vi "S2DS_IncorporateUnitsinChannelNames.vi"(5 "User info":string[](array[string]), 9 "All channel parameters (in)":T1 {"Scan parameters"."Y data taking" items=["in both direction", "in up direction only", "in down direction only"]; "Scan parameters"."X data taking" items=["in both direction", "in up direction only", "in down direction only"]}) -> (3 "All channel info (out)":T10)   [LabVIEW 2025]
uses:
  TYPE DEFS/S2DS_Display info.ctl
  TYPE DEFS/S2DS_All Channel Parameters.ctl
  TYPE DEFS/S2DS_WC info.ctl
  TYPE DEFS/S2DS_Single WC info.ctl
  TYPE DEFS/S2DS_RC info.ctl
  TYPE DEFS/S2DS_Single RC info.ctl
  TYPE DEFS/S2DS_DAC info new.ctl
  TYPE DEFS/S2DS_Single DC info.ctl
  TYPE DEFS/S2DS_Array Inst Info.ctl
  TYPE DEFS/S2DS_Sweep Info.ctl
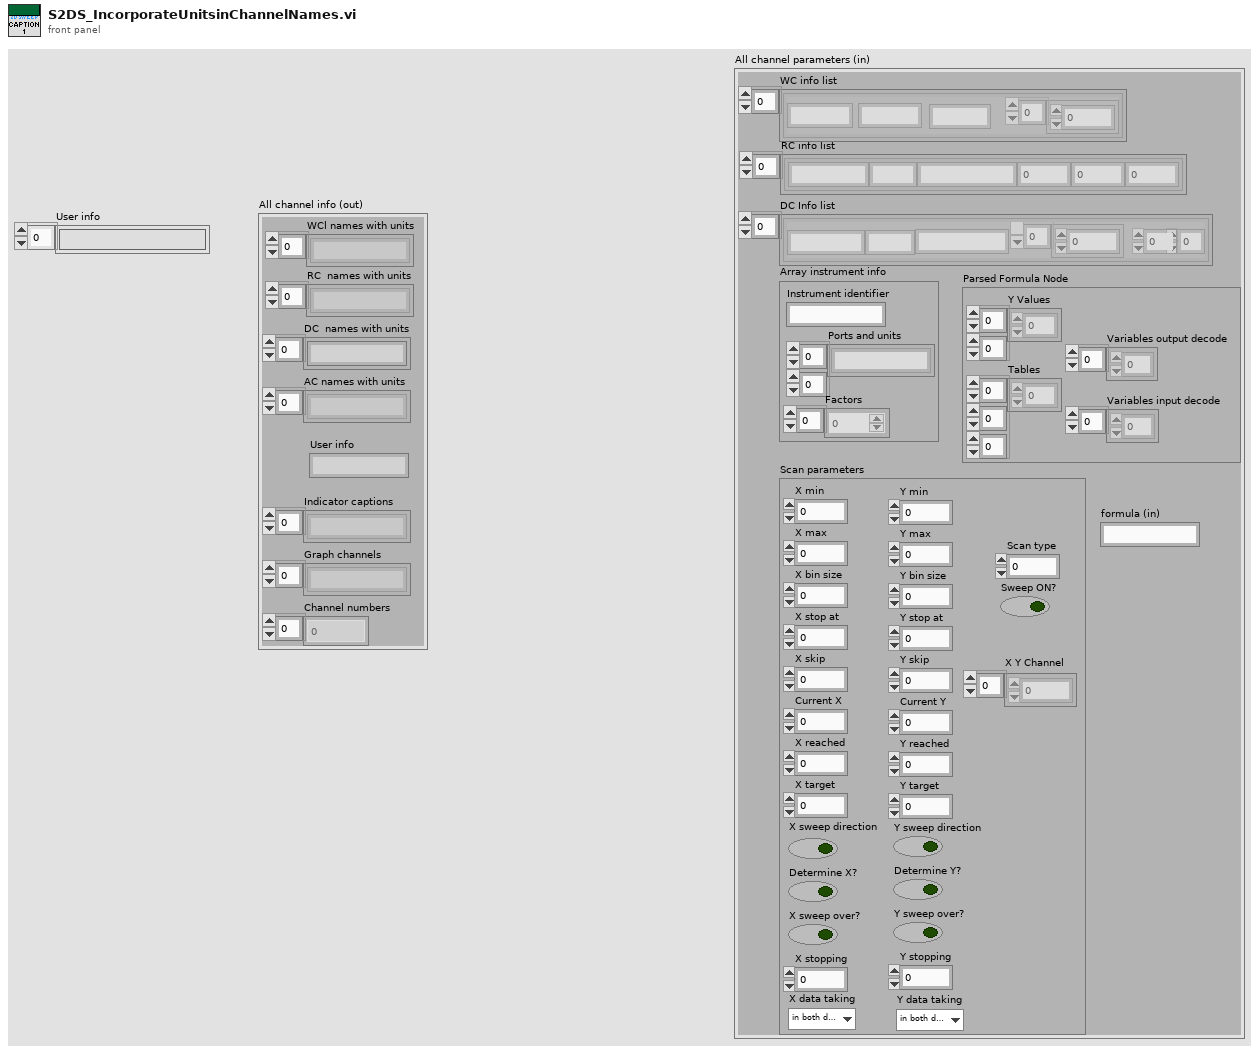
[diagram p1: front panel]
types:
  T1 = typedef "S2DS_All Channel Parameters.ctl" = cluster{"WC info list":T2, "RC info list":T4, "DC Info list":T6, "Array instrument info":T8, "Scan parameters":T9, "Parsed Formula Node":cluster{"Y Values":dbl[][], "Tables":i32[][][], "Variables input decode":i32[], "Variables output decode":i32[]}, "formula (in)":string}
  T2 = typedef "S2DS_WC info.ctl" = T3[]
  T3 = typedef "S2DS_Single WC info.ctl" = cluster{"Instrument identifier":string, "Write channel parameters":dbl[], "Name":string, "Unit":string}
  T4 = typedef "S2DS_RC info.ctl" = T5[]
  T5 = typedef "S2DS_Single RC info.ctl" = cluster{"Instrument identifier":string, "Factor":dbl, "Averaging":i32, "Wait (ms)":i32, "Unit":string, "Name":string}
  T6 = typedef "S2DS_DAC info new.ctl" = T7[]
  T7 = typedef "S2DS_Single DC info.ctl" = cluster{"Operation identifier":string, "DC parameters":dbl[], "U":i32, "V":i32, "Name":string, "Unit":string}
  T8 = typedef "S2DS_Array Inst Info.ctl" = cluster{"Instrument identifier":string, "Ports and units":string[][], "Factors":dbl[]}
  T9 = typedef "S2DS_Sweep Info.ctl" = cluster{"X min":ext, "X max":dbl, "Y min":dbl, "Y max":dbl, "X bin size":dbl, "Y bin size":dbl, "X stop at":dbl, "Y stop at":dbl, "X skip":u64, "Y skip":u64, "Current X":dbl, "Current Y":dbl, "X reached":i32, "Y reached":i32, "X target":dbl, "Y target":dbl, "Sweep ON?":bool, "X sweep direction":bool, "Y sweep direction":bool, "Determine X?":bool, "Determine Y?":bool, "X sweep over?":bool, "Y sweep over?":bool, "Scan type":i32, "X stopping":i32, "Y stopping":i32, "X Y Channel":u16[], "X data taking":u16, "Y data taking":u16}
  T10 = typedef "S2DS_Display info.ctl" = cluster{"WCl names with units":string[], "RC  names with units":string[], "DC  names with units":string[], "AC names with units":string[], "Indicator captions":string[], "Graph channels":string[], "Channel numbers":i32[], "User info":string}
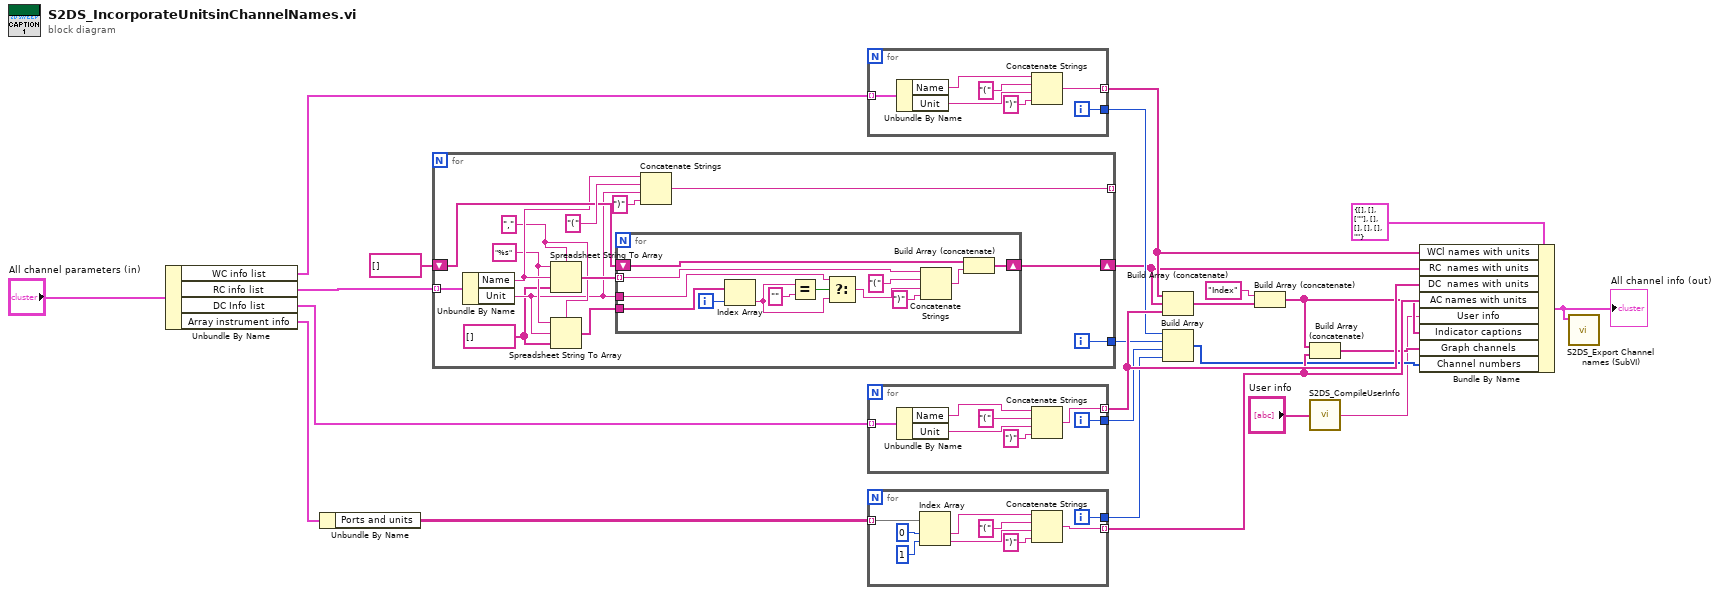
[diagram p0: block diagram]
diagram:
  n1 = Unbundle By Name("All channel parameters (in)") -> ("WC info list"=w7:T2, "RC info list"=w6:T4, "DC Info list"=w5:T6, "Array instrument info"=w4:T8)
  n2 = Unbundle By Name(w4) -> ("Ports and units"=w3:string[][])
  n3 = for {
    tunnel: w6 -> [w35] mode=indexing
    tunnel: [w34] -> _ mode=indexing
    tunnel: [w36] -> w18
    shift-right: [w31] -> w1
    shift-left: string[] [] -> [w32]
    i -> [w36]
    w26 = string[] []
    w29 = "," ("delimiter (Tab)")
    w28 = "%s" ("format string")
    n4 = Unbundle By Name(w35) -> ("Name"=w30:string, "Unit"=w27:string)
    n5 = Spreadsheet String To Array(delimiter (Tab)=w29, format string=w28, spreadsheet string=w30, array type (2D Dbl)=w26) -> (array=w33:string[])
    n6 = Spreadsheet String To Array(delimiter (Tab)=w29, format string=w28, spreadsheet string=w27, array type (2D Dbl)=w26) -> (array=w25:string[])
    n7 = for {
      tunnel: w33 -> [w51] mode=indexing
      tunnel: w27 -> [w41]
      shift-right: [w46] -> w31
      shift-left: w32 -> [w47]
      tunnel: w25 -> [w45]
      i -> [w44]
      n8 = Index Array(array=w45, index=w44) -> (element=w40:string)
      n9 = Equal?(x=w40, y="") -> (x = y?=w42:bool)
      n10 = Select(t=w41, s=w42, f=w40) -> (s? t:f=w39:string)
      n11 = Concatenate Strings(w51, "(" ("string"), w39, ")" ("string")) -> (w48:string)
      n12 = Build Array (concatenate)(w47, w48) -> (w46:string[])
    }
    n13 = Concatenate Strings(w30, "(" ("string"), w27, ")" ("string")) -> (w34:string)
  }
  n14 = for {
    tunnel: w7 -> [w54] mode=indexing
    tunnel: [w56] -> w23 mode=indexing
    tunnel: [w55] -> w19
    i -> [w55]
    n15 = Unbundle By Name(w54) -> ("Name"=w53:string, "Unit"=w52:string)
    n16 = Concatenate Strings(w53, "(" ("string"), w52, ")" ("string")) -> (w56:string)
  }
  n17 = for {
    tunnel: w5 -> [w61] mode=indexing
    tunnel: [w63] -> w22 mode=indexing
    tunnel: [w62] -> w17
    i -> [w62]
    n18 = Unbundle By Name(w61) -> ("Name"=w60:string, "Unit"=w59:string)
    n19 = Concatenate Strings(w60, "(" ("string"), w59, ")" ("string")) -> (w63:string)
  }
  n20 = for {
    tunnel: w3 -> [w74] mode=indexing
    tunnel: [w67] -> w21 mode=indexing
    tunnel: [w66] -> w16
    i -> [w66]
    n21 = Index Array(array=w74, index #1=0 ("index"), index #2=1 ("index")) -> (element #1=w71:string, element #2=w69:string)
    n22 = Concatenate Strings(w71, "(" ("string"), w69, ")" ("string")) -> (w67:string)
  }
  n23 = Build Array (concatenate)(w23, w1, w22) -> (w11:string[])
  n24 = Build Array(w19, w18, w17, w16) -> (w15:i32[])
  n25 = Build Array (concatenate)("Index", w11) -> (w13:string[])
  n26 = Build Array (concatenate)(w13, w21) -> (w20:string[])
  n27 = call "S2DS_CompileUserInfo.vi"("User info"="User info") -> ("String"=w10:string)
  n28 = Bundle By Name(cluster=T10 {"WCl names with units"=[], "RC  names with units"=[], "DC  names with units"=[""], "AC names with units"=[], "Indicator captions"=[], "Graph channels"=[], "Channel numbers"=[], "User info"=""} ("All channel info (out)"), "WCl names with units"=w23, "RC  names with units"=w1, "DC  names with units"=w22, "AC names with units"=w21, "User info"=w10, "Indicator captions"=w13, "Graph channels"=w20, "Channel numbers"=w15) -> (w14:T10)
  "All channel info (out)" <- w14
  n29 = call "S2DS_Export Channel names (SubVI).vi"("All channel info (in)"=w14) -> ()  [unwired: 10 in, 1 out]
